vi "OldClimbSetSensorPoseRight.vi"(11 "ClimbSetSensorPoseRight":dbl) -> ()   [LabVIEW 2023]
uses:
  OldClimbGlobal.vi
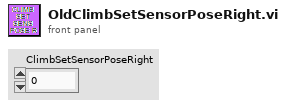
[diagram p1: front panel]
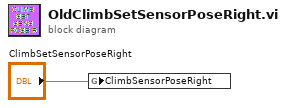
[diagram p0: block diagram]
diagram:
  n1 = global write "OldClimbGlobal.vi" "ClimbSensorPoseRight"("ClimbSetSensorPoseRight") -> ()
